vi "Select Ball By Confidence.vi"(10 "Array":T1[](array[typedef]) {"robots_blue"."height" format="%+4.3f"; "robots_blue"."pixel_y" format="%+4.3f"; "robots_blue"."pixel_x" format="%+4.3f"; "robots_blue"."orientation" format="%+4.3f"; "robots_blue"."y" format="%+4.3f"; "robots_blue"."confidence" format="%4.3f"; "robots_blue"."x" format="%+4.3f"; "robots_yellow"."height" format="%+4.3f"; "robots_yellow"."pixel_y" format="%+4.3f"; "robots_yellow"."pixel_x" format="%+4.3f"; "robots_yellow"."orientation" format="%+4.3f"; "robots_yellow"."y" format="%+4.3f"; "robots_yellow"."confidence" format="%4.3f"; "robots_yellow"."x" format="%+4.3f"}, 11 "balls":T4[](array[typedef])) -> (3 "balls out":T4[](array[typedef]))   [LabVIEW 2017]
uses:
  SSL Detection Ball.ctl
  <vilib>/Analysis/Matrix/Datatypes/RealMatrix.ctl
  SSL Detection Frame.ctl
  SSL Detection Robot.ctl
  <vilib>/Analysis/Matrix/NI_Matrix.lvlib
panel:
  in  "Boolean":bool
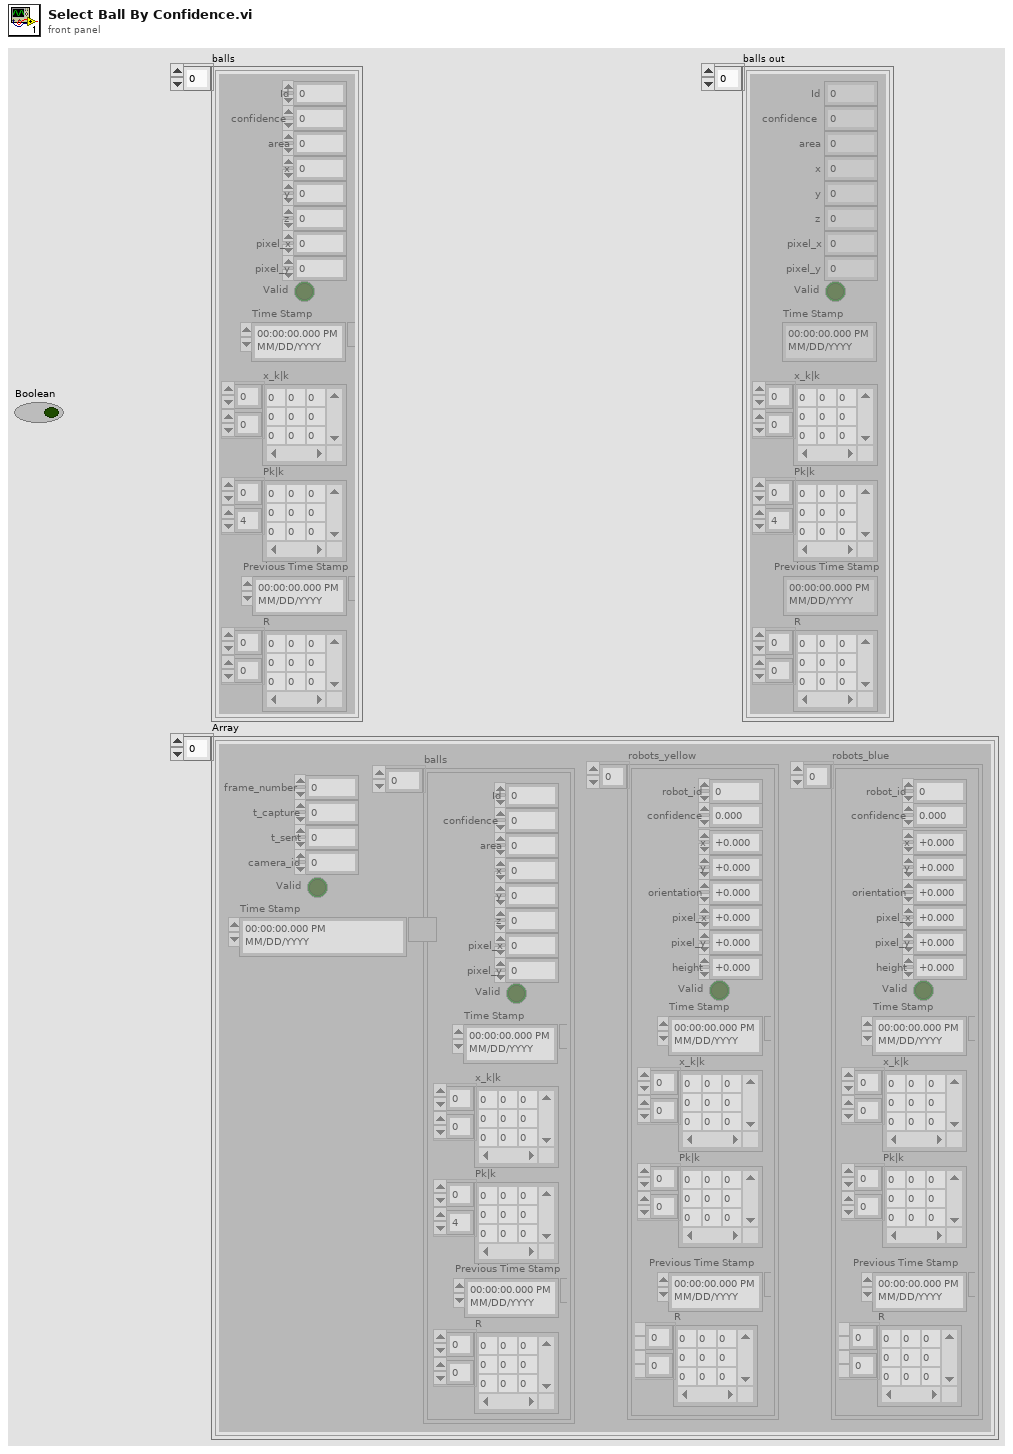
[diagram p1: front panel]
types:
  T1 = typedef "SSL Detection Frame.ctl" = cluster{"frame_number":u32, "t_capture":dbl, "t_sent":dbl, "camera_id":u32, "robots_yellow":T2[], "robots_blue":T2[], "balls":T4[], "Valid":bool, "Time Stamp":timestamp}
  T2 = typedef "SSL Detection Robot.ctl" = cluster{"x":sgl, "robot_id":u32, "confidence":sgl, "y":sgl, "orientation":sgl, "pixel_x":sgl, "pixel_y":sgl, "height":sgl, "Valid":bool, "Time Stamp":timestamp, "x_k|k":T3, "Pk|k":T3, "Previous Time Stamp":timestamp, "R":T3}
  T3 = typedef "NI_Matrix.lvlib/RealMatrix.ctl" = dbl[][]
  T4 = typedef "SSL Detection Ball.ctl" = cluster{"x":sgl, "area":u32, "confidence":sgl, "y":sgl, "z":sgl, "pixel_x":sgl, "pixel_y":sgl, "Valid":bool, "Time Stamp":timestamp, "x_k|k":T3, "Pk|k":T3, "Id":u32, "Previous Time Stamp":timestamp, "R":T3}
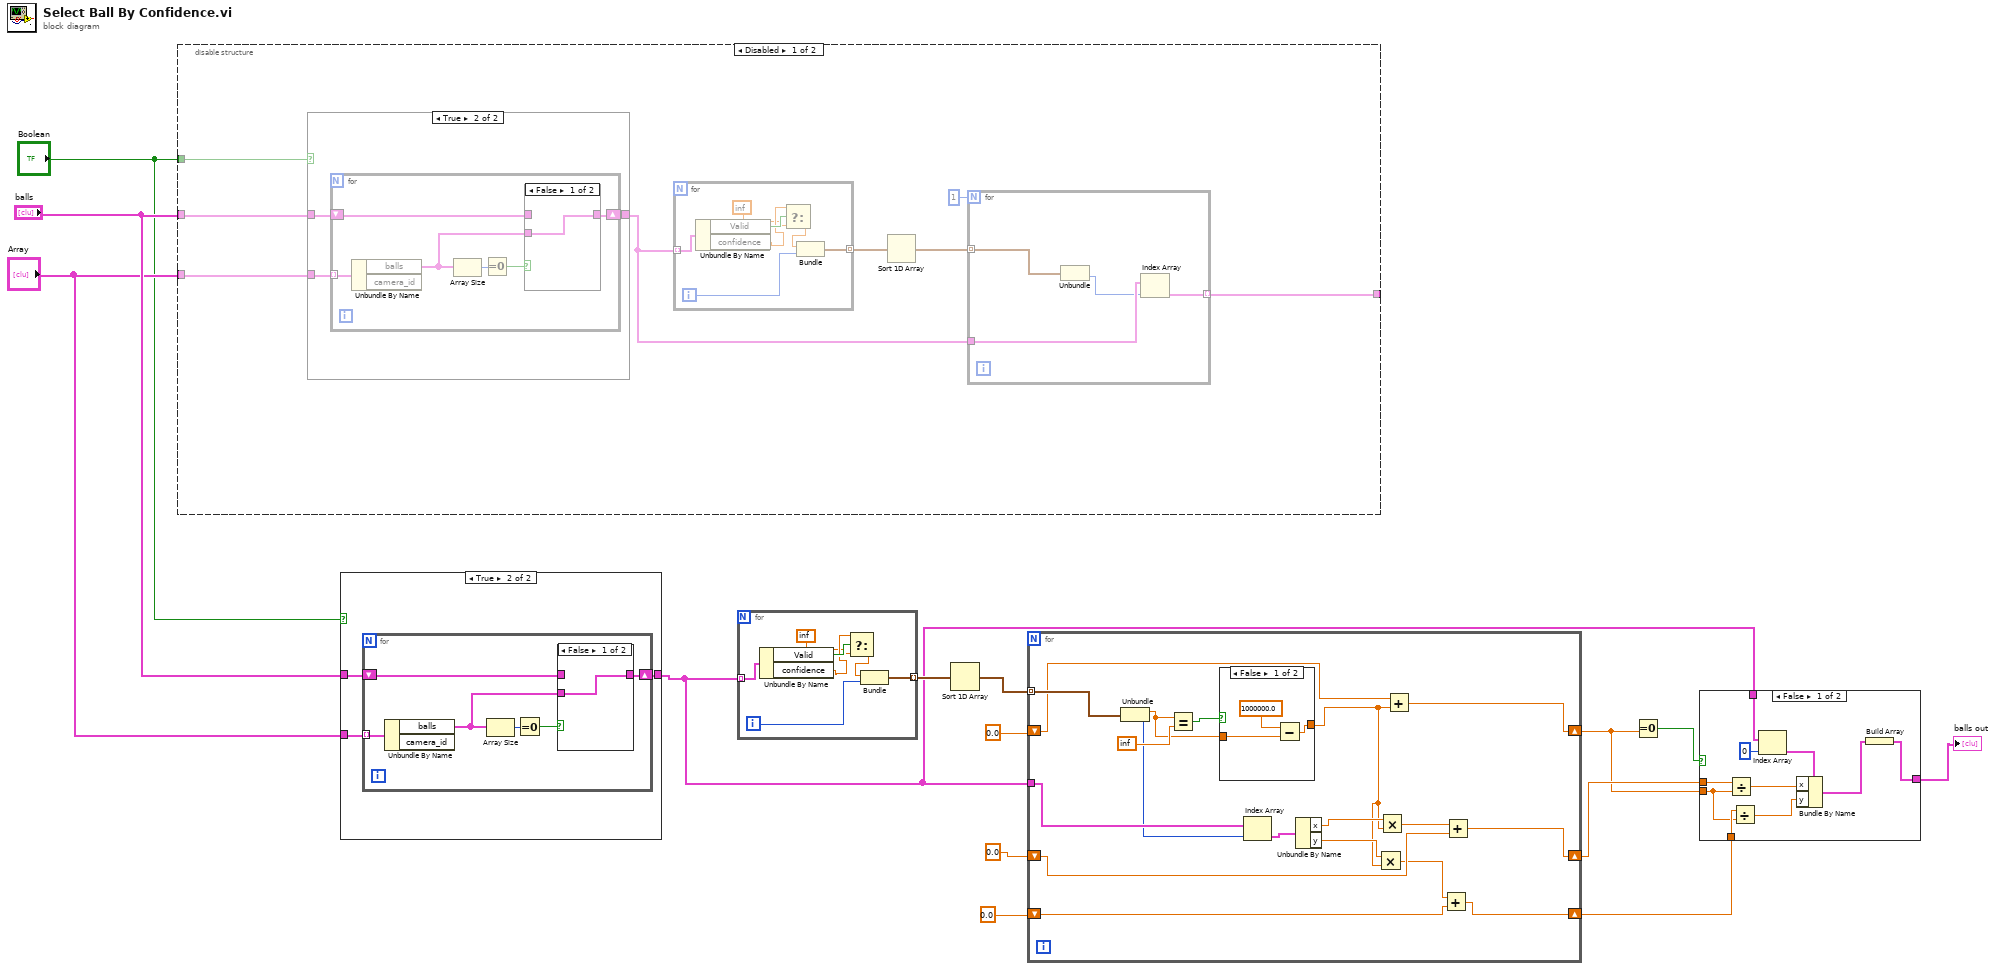
[diagram p0: block diagram]
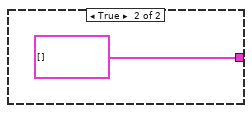
[diagram p2: hidden frame]
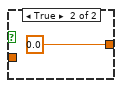
[diagram p3: hidden frame]
diagram:
  n1 = disable-structure shown="Disabled" {
    disable-tunnel: [w20 _] -> _
    disable-tunnel: "Array" -> [w18 _]
    disable-tunnel: "balls" -> [w16 _]
    disable-tunnel: "Boolean" -> [w15 _]
    frame Disabled {
      n2 = case shown="True" w15 {
        tunnel: w18 -> [_ w26]
        tunnel: [w23 w25] -> w17
        tunnel: w16 -> [w23 w24]
        frame False {
        }
        frame True {
          n3 = for {
            tunnel: w26 -> [w32] mode=indexing
            shift-right: [w29] -> w25
            shift-left: w24 -> [w27]
            n4 = Unbundle By Name(w32) -> ("balls"=w28:T4[])  [unwired: 1 out]
            n5 = Array Size(array=w28) -> (size(s)=w31:i32)
            n6 = Equal To 0?(x=w31) -> (x = 0?=w30:bool)
            n7 = case shown="False" w30 {
              tunnel: [w33 w34] -> w29
              tunnel: w28 -> [w33 _]
              tunnel: w27 -> [_ w34]
              frame False {
              }
              frame True {
              }
            }
          }
        }
      }
      n8 = for {
        tunnel: w17 -> [w45] mode=indexing
        tunnel: [w44] -> w22 mode=indexing
        i -> [w43]
        n9 = Unbundle By Name(w45) -> ("Valid"=w42:bool, "confidence"=w41:sgl)
        n10 = Select(t=w41, s=w42, f=inf) -> (s? t:f=w40:dbl)
        n11 = Bundle("confidence"=w40, w43) -> (w44:cluster{"confidence":dbl, i32})  [unwired: 1 in]
      }
      n12 = Sort 1D Array(array=w22) -> (sorted array=w21:cluster{"confidence":dbl, i32}[])
      n13 = for {
        N: 1 -> [_]
        tunnel: w21 -> [w38] mode=indexing
        tunnel: w17 -> [w37]
        tunnel: [w35] -> w20 mode=indexing
        n14 = Unbundle(w38) -> (w36:i32)  [unwired: 1 out]
        n15 = Index Array(array=w37, index=w36) -> (element=w35:T4)
      }
    }
    frame Enabled {
    }
  }
  n16 = case shown="True" "Boolean" {
    tunnel: "Array" -> [_ w49]
    tunnel: [w46 w48] -> w5
    tunnel: "balls" -> [w46 w47]
    frame False {
    }
    frame True {
      n17 = for {
        tunnel: w49 -> [w55] mode=indexing
        shift-right: [w52] -> w48
        shift-left: w47 -> [w50]
        n18 = Unbundle By Name(w55) -> ("balls"=w51:T4[])  [unwired: 1 out]
        n19 = Array Size(array=w51) -> (size(s)=w54:i32)
        n20 = Equal To 0?(x=w54) -> (x = 0?=w53:bool)
        n21 = case shown="False" w53 {
          tunnel: [w56 w57] -> w52
          tunnel: w51 -> [w56 _]
          tunnel: w50 -> [_ w57]
          frame False {
          }
          frame True {
          }
        }
      }
    }
  }
  n22 = for {
    tunnel: w5 -> [w64] mode=indexing
    tunnel: [w63] -> w11 mode=indexing
    i -> [w62]
    n23 = Unbundle By Name(w64) -> ("Valid"=w61:bool, "confidence"=w60:sgl)
    n24 = Select(t=w60, s=w61, f=inf) -> (s? t:f=w59:dbl)
    n25 = Bundle("confidence"=w59, w62) -> (w63:cluster{"confidence":dbl, i32})  [unwired: 1 in]
  }
  n26 = Sort 1D Array(array=w11) -> (sorted array=w10:cluster{"confidence":dbl, i32}[])
  n27 = for {
    tunnel: w10 -> [w82] mode=indexing
    tunnel: w5 -> [w78]
    shift-right: [w74] -> w2
    shift-left: 0.0 -> [w75]
    shift-right: [w68] -> w3
    shift-left: 0.0 -> [w69]
    shift-right: [w65] -> w1
    shift-left: 0.0 -> [w66]
    n28 = Unbundle(w82) -> ("confidence"=w79:dbl, w77:i32)
    n29 = Equal?(x=w79, y=inf) -> (x = y?=w80:bool)
    n30 = case shown="False" w80 {
      tunnel: [w83 0.0] -> w71
      tunnel: w79 -> [w84 _]
      frame False {
        n31 = Subtract(x=1000000.0, y=w84) -> (x-y=w83:dbl)
      }
      frame True {
      }
    }
    n32 = Index Array(array=w78, index=w77) -> (element=w76:T4)
    n33 = Unbundle By Name(w76) -> ("x"=w73:sgl, "y"=w72:sgl)
    n34 = Multiply(x=w72, y=w71) -> (x*y=w67:dbl)
    n35 = Multiply(x=w73, y=w71) -> (x*y=w70:dbl)
    n36 = Add(x=w75, y=w71) -> (x+y=w74:dbl)
    n37 = Add(x=w67, y=w66) -> (x+y=w65:dbl)
    n38 = Add(x=w70, y=w69) -> (x+y=w68:dbl)
  }
  n39 = Equal To 0?(x=w2) -> (x = 0?=w6:bool)
  n40 = case shown="False" w6 {
    tunnel: w5 -> [w96 _]
    tunnel: [w92 T4[] [] ("balls out")] -> w4
    tunnel: w3 -> [w91 _]
    tunnel: w2 -> [w88 _]
    tunnel: w1 -> [w89 _]
    frame False {
      n41 = Divide(x=w91, y=w88) -> (x/y=w90:dbl)
      n42 = Divide(x=w89, y=w88) -> (x/y=w87:dbl)
      n43 = Index Array(array=w96, index=0) -> (element=w94:T4)
      n44 = Bundle By Name(cluster=w94, "x"=w90, "y"=w87) -> (w93:T4)
      n45 = Build Array(w93) -> (w92:T4[])
    }
    frame True {
    }
  }
  "balls out" <- w4
